vi "Database_search.vi"() -> ()   [LabVIEW 2021]
doc: "This VI search the data in the data base."
uses:
  Controls/Acc-data-array-of-cluster.ctl
  Controls/Search_option.ctl
panel:
  in  "Stop":bool
  out "Valid Upto Search Result":T1[](array[typedef])
  out "Card Number Search Result":T1
  out "Card Holder Name Search result":T1[](array[typedef])
  out "Search Time (ms)":dbl
  in  "Search Option":T2
  in  "Valid Upto":dbl=2010.0 min=2000.0 max=2065.0 step=1.0
  in  "Card Number":dbl
  in  "Card Holder Name":string
  in  "Account Details":T1[](array[typedef])=[{"Card Number"=11.0, "Valid Upto"=2050.0, "Card Holder Name"="Tom"}, {"Card Number"=12.0, "Valid Upto"=2024.0, "Card Holder Name"="Jerry"}, {"Card Number"=110.0, "Valid Upto"=2050.0, "Card Holder Name"="Jerry"}]
  # "DATA BASE"
  # "SEARCH BOX"
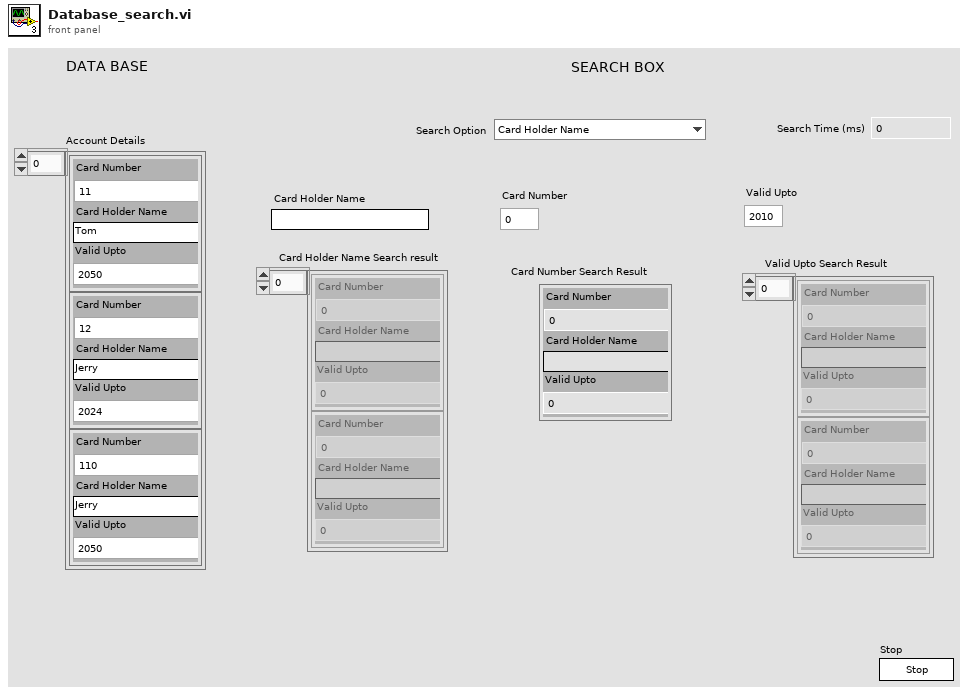
[diagram p1: front panel]
types:
  T1 = typedef "Acc-data-array-of-cluster.ctl" = cluster{"Card Number":dbl, "Valid Upto":dbl, "Card Holder Name":string}
  T2 = typedef "Search_option.ctl" = enum16{"Card Holder Name ", "Card Number", "Valid Upto"}
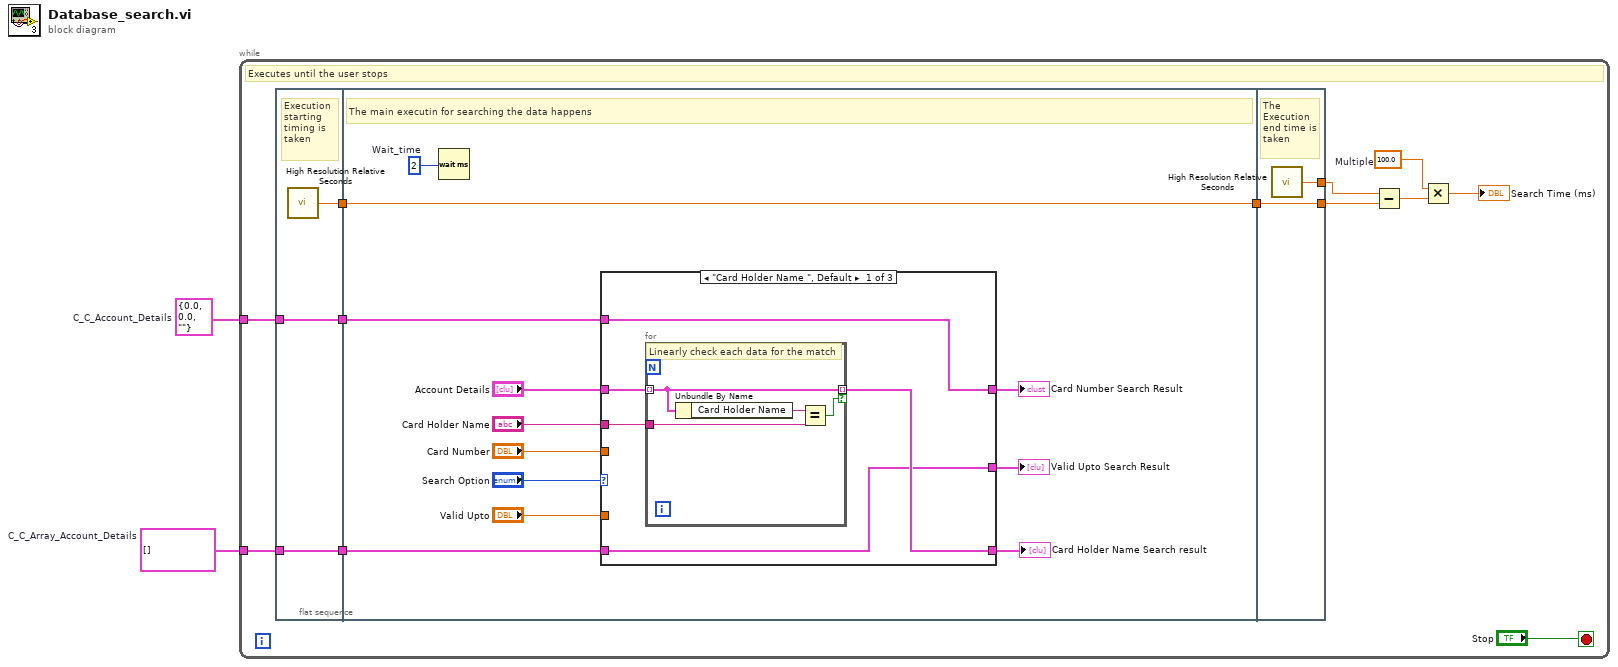
[diagram p0: block diagram]
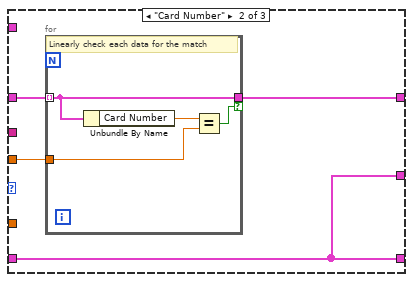
[diagram p2: hidden frame]
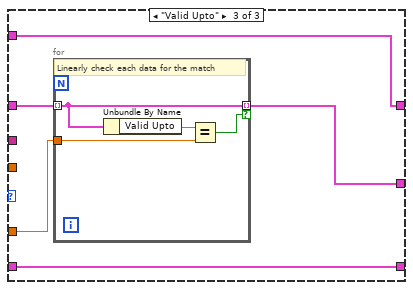
[diagram p3: hidden frame]
diagram:
  w2 = T1 {"Card Number"=0.0, "Valid Upto"=0.0, "Card Holder Name"=""}  # C_C_Account_Details
  w1 = T1[] []  # C_C_Array_Account_Details
  n1 = while {
    tunnel: w2 -> [w7]
    tunnel: w1 -> [w5]
    stop <- "Stop" stop-if-true
    w3 = 100.0  # Multiple
    # "Executes until the user stops"
    n2 = flat-sequence {
      tunnel: [w17] -> w14
      tunnel: [w16] -> w8
      tunnel: w7 -> [w16]
      tunnel: [w15] -> w6
      tunnel: w5 -> [w15]
      tunnel: w14 -> [w22]
      tunnel: [w22] -> w9
      tunnel: w8 -> [w19]
      tunnel: w6 -> [w18]
      tunnel: [w56] -> w12
      tunnel: [w57] -> w13
      tunnel: w9 -> [w57]
      frame #0 {
        # "Execution starting timing is  taken"
        n3 = call <vilib>:"High Resolution Relative Seconds.vi"() -> ("relative seconds"=w17:dbl)
      }
      frame #1 {
        w21 = u32 2  # Wait_time
        # "The main executin for searching the data happens"
        n4 = Wait (ms)(milliseconds to wait=w21) -> ()  [unwired: 1 out]
        n5 = case shown="\"Card Holder Name \", Default" "Search Option" {
          tunnel: "Account Details" -> [w34 w40 w51]
          tunnel: "Card Number" -> [_ w42 _]
          tunnel: [w31 w41 w48] -> w20
          tunnel: "Card Holder Name" -> [w33 _ _]
          tunnel: [w32 w39 w47] -> w25
          tunnel: "Valid Upto" -> [_ _ w50]
          tunnel: [w30 w39 w49] -> w23
          tunnel: w19 -> [w31 _ w48]
          tunnel: w18 -> [w30 w39 w47]
          frame "Card Holder Name ", Default {
            n6 = for {
              tunnel: [w36] -> w32 mode=indexing if=w37
              tunnel: w34 -> [w36] mode=indexing
              tunnel: w33 -> [w35]
              # "Linearly check each data for the match"
              n7 = Unbundle By Name(w36) -> ("Card Holder Name"=w38:string)
              n8 = Equal?(x=w38, y=w35) -> (x = y?=w37:bool)
            }
          }
          frame "Card Number" {
            n9 = for {
              tunnel: w42 -> [w45]
              tunnel: [w43] -> w41 if=w44
              tunnel: w40 -> [w43] mode=indexing
              # "Linearly check each data for the match"
              n10 = Unbundle By Name(w43) -> ("Card Number"=w46:dbl)
              n11 = Equal?(x=w46, y=w45) -> (x = y?=w44:bool)
            }
          }
          frame "Valid Upto" {
            n12 = for {
              tunnel: [w53] -> w49 mode=indexing if=w54
              tunnel: w51 -> [w53] mode=indexing
              tunnel: w50 -> [w52]
              # "Linearly check each data for the match"
              n13 = Unbundle By Name(w53) -> ("Valid Upto"=w55:dbl)
              n14 = Equal?(x=w55, y=w52) -> (x = y?=w54:bool)
            }
          }
        }
        "Card Holder Name Search result" <- w25
        "Card Number Search Result" <- w20
        "Valid Upto Search Result" <- w23
      }
      frame #2 {
        # "The Execution end time is taken"
        n15 = call <vilib>:"High Resolution Relative Seconds.vi"() -> ("relative seconds"=w56:dbl)
      }
    }
    n16 = Subtract(x=w12, y=w13) -> (x-y=w11:dbl)
    n17 = Multiply(x=w3, y=w11) -> (x*y=→"Search Time (ms)":dbl)
  }
